vi "Dot Net Memory Magic.vi"(8 "error in (no error)":errorcluster) -> (0 "error out":errorcluster, 3 "Private Memory (MB)":sgl)   [LabVIEW 2019]
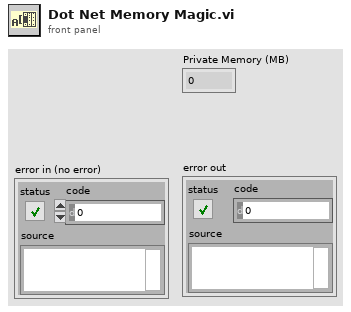
[diagram p1: front panel]
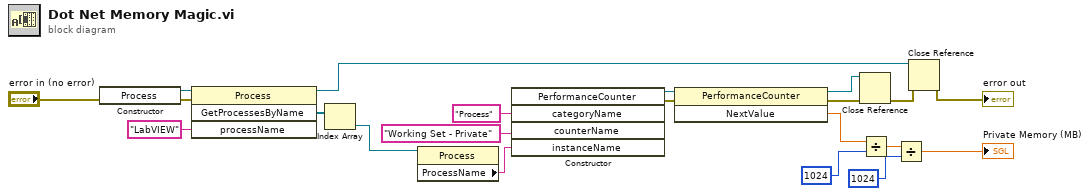
[diagram p0: block diagram]
diagram:
  n1 = constructor class="Process"(error in="error in (no error)") -> (reference out=w20:refnum<k24>, error out=w21:errorcluster)  [unwired: 2 in, 1 out]
  n2 = invoke class="Process" method="GetProcessesByName"(reference=w20, error in=w21, "processName"="LabVIEW" ("counterName")) -> (reference out=w9:refnum<k24>, "GetProcessesByName"=w14:refnum<k24>[])  [unwired: 1 in, 2 out]
  n3 = Index Array(array=w14) -> (element=w13:refnum<k24>)  [unwired: 1 in]
  n4 = property class="Process"(reference=w13) -> ("ProcessName"=w15:string)  [unwired: 1 in, 2 out]
  n5 = constructor class="PerformanceCounter"("categoryName"="Process", "counterName"="Working Set - Private", "instanceName"=w15) -> (reference out=w16:refnum<k24>, error out=w17:errorcluster)  [unwired: 3 in, 4 out]
  n6 = invoke class="PerformanceCounter" method="NextValue"(reference=w16, error in=w17) -> (reference out=w10:refnum<k24>, error out=w11:errorcluster, "NextValue"=w6:sgl)  [unwired: 1 in]
  n7 = Close Reference(reference=w10, error in (no error)=w11) -> (error out=w8:errorcluster)
  n8 = Divide(x=w6, y=i64 1024) -> (x/y=w4:sgl)
  n9 = Divide(x=w4, y=i64 1024) -> (x/y=→"Private Memory (MB)":sgl)
  n10 = Close Reference(reference=w9, error in (no error)=w8) -> (error out=→"error out":errorcluster)
